vi "String-to-num.vi"(2 "error in (no error)":errorcluster, 3 "Value_String":string[](array[string])) -> (0 "error out":errorcluster, 1 "Value_Num":dbl[](array[numeric]))   [LabVIEW 2014]
doc: "This VI takes the Decimal string array as an input and converts it into an array of double.\n\nDesigned by HB\nhaba@dtu.dk"
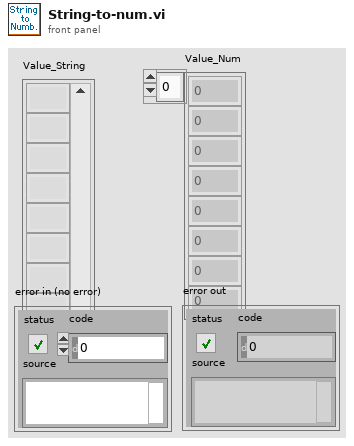
[diagram p1: front panel]
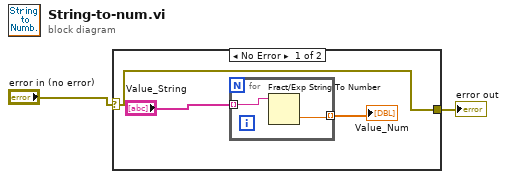
[diagram p0: block diagram]
diagram:
  n1 = case shown="No Error" "error in (no error)" {
    selector: "error in (no error)" -> [w3 w8]
    tunnel: [w3 w8] -> w1
    frame No Error {
      n2 = for {
        tunnel: "Value_String" -> [w7] mode=indexing
        tunnel: [w6] -> w4 mode=indexing
        n3 = Fract/Exp String To Number(string=w7) -> (number=w6:dbl)  [unwired: 3 in, 1 out]
      }
      "Value_Num" <- w4
    }
    frame Error {
    }
  }
  "error out" <- w1
